vi "Resample (constant to constant,single -channel).vi"(5 "anti-aliasing?":bool=TRUE, 6 "FIR filter specifications":T1={"alias rejection (dB)"=120.0, "normalized bandwidth"=0.4536} {"normalized bandwidth" format="%.4f"; "alias rejection (dB)" format="%.2f"}, 7 "reset?":bool, 8 "error in (no error)":errorcluster, 9 "dt":dbl=1.0, 10 "delay":dbl, 11 "X":dbl[](array[numeric])) -> (0 "error out":errorcluster, 2 "t0":dbl, 3 "Y":dbl[](array[numeric]) format="%#.6g")   [LabVIEW 2020, in "NI_AALPro.lvlib"]
doc: "Resamples input signal <B>X</B> according to <B>delay</B> and <B>dt</B> using an FIR filter implementation. Wire data to the <B>X</B> input to determine the polymorphic instance to use or manually select the instance."
uses:
  NI_AALPro.lvlib
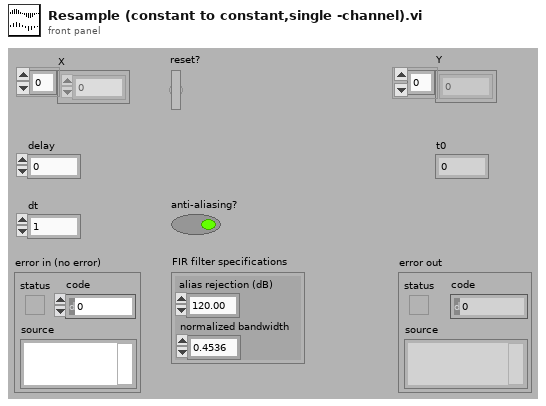
[diagram p1: front panel]
types:
  T1 = cluster{"alias rejection (dB)":dbl, "normalized bandwidth":dbl}
  T2 = cluster{"new sample period":dbl, "Timing Jitter":enum32{"Interpolation", "Rounding"}, "first point location":dbl, "prototype filter":cluster{"h":dbl[], "Max Decimation":i32}}
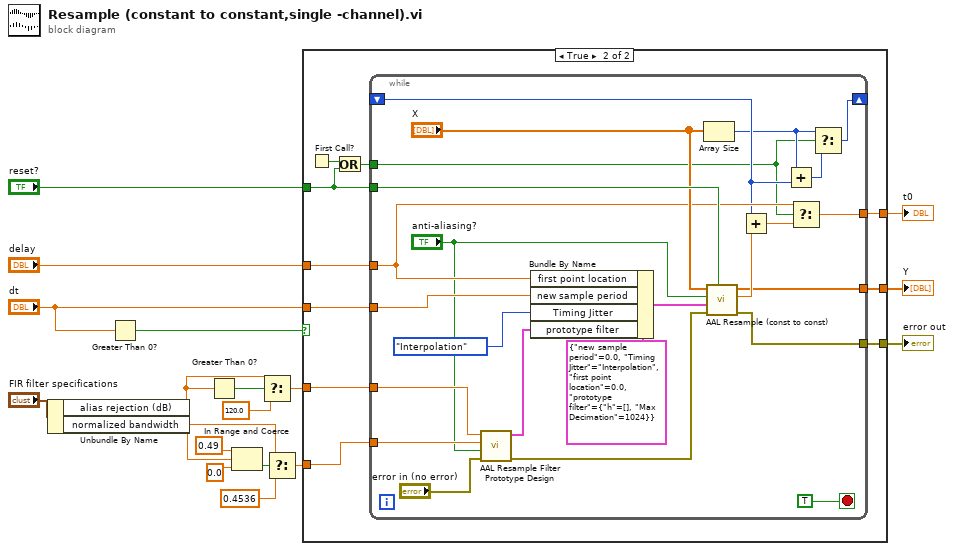
[diagram p0: block diagram]
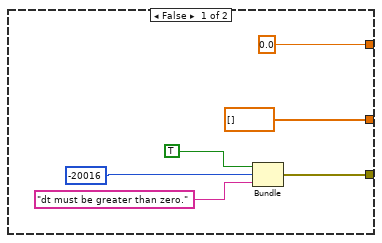
[diagram p2: hidden frame]
diagram:
  n1 = Unbundle By Name("FIR filter specifications") -> ("alias rejection (dB)"=w1:dbl, "normalized bandwidth"=w5:dbl)
  n2 = Greater Than 0?(x="dt") -> (x > 0?=w13:bool)
  n3 = Greater Than 0?(x=w1) -> (x > 0?=w2:bool)
  n4 = In Range and Coerce(upper limit=0.49, x=w5, lower limit=0.0 ("upper limit")) -> (In Range?=w6:bool)  [unwired: 1 out]
  n5 = Select(t=w1, s=w2, f=120.0) -> (s? t:f=w7:dbl)
  n6 = Select(t=w5, s=w6, f=0.4536 ("upper limit")) -> (s? t:f=w3:dbl)
  n7 = case shown="True" w13 {
    tunnel: "delay" -> [_ w34]
    tunnel: "reset?" -> [_ w32]
    tunnel: [0.0 ("delay") w30] -> w16
    tunnel: [dbl[] [] ("Y") w29] -> w15
    tunnel: [w22 w28] -> w14
    tunnel: "dt" -> [_ w27]
    tunnel: w7 -> [_ w26]
    tunnel: w3 -> [_ w25]
    frame False {
      n8 = Bundle(TRUE, "DtGTZeroErr"=-20016, "dt must be greater than zero.") -> (w22:cluster{bool, "DtGTZeroErr":i32, string})  [unwired: 1 in]
    }
    frame True {
      n9 = First Call?() -> (First Call?: T/F=w31:bool)
      n10 = Or(x=w31, y=w32) -> (x .or. y?=w33:bool)
      n11 = while {
        shift-right: [w47] -> _
        shift-left: _ -> [w44]
        tunnel: w32 -> [w52]
        tunnel: w34 -> [w45]
        tunnel: w33 -> [w42]
        tunnel: [w41] -> w30
        tunnel: [w40] -> w29
        tunnel: [w39] -> w28
        tunnel: w27 -> [w38]
        tunnel: w26 -> [w37]
        tunnel: w25 -> [w36]
        stop <- TRUE stop-if-true
        n12 = call "AAL Resample Filter Prototype Design.vi"("error in (no error)"="error in (no error)", "alias free"="anti-aliasing?", "normalized bandwidth"=w36, "A stop [dB]"=w37) -> ("error out"=w57:errorcluster, "filter prototype"=w54:cluster{"coefficients":dbl[], "factor":i32})  [unwired: 5 in, 1 out]
        n13 = Bundle By Name(cluster=T2 {"new sample period"=0.0, "Timing Jitter"=enum."Interpolation", "first point location"=0.0, "prototype filter"={"h"=[], "Max Decimation"=1024}} ("config"), "first point location"=w45, "new sample period"=w38, "Timing Jitter"=enum32{"Interpolation", "Rounding"}."Interpolation" ("timing jitter"), "prototype filter"=w54) -> (w53:T2)
        n14 = Array Size(array="X") -> (size(s)=w43:i32)
        n15 = call "AAL Resample (const to const).vi"("reset?"=w52, "error in (no error)"=w57, "config"=w53, "anti-aliasing?"="anti-aliasing?", "X"="X") -> ("error out"=w39:errorcluster, "normalized t0"=w49:dbl, "Y"=w40:dbl[])  [unwired: 4 in]
        n16 = Add(x=w44, y=w49) -> (x+y=w48:dbl)
        n17 = Add(x=w43, y=w44) -> (x+y=w46:i32)
        n18 = Select(t=w45, s=w42, f=w48) -> (s? t:f=w41:dbl)
        n19 = Select(t=w43, s=w42, f=w46) -> (s? t:f=w47:i32)
      }
    }
  }
  "t0" <- w16
  "Y" <- w15
  "error out" <- w14
